vi "Poll Caller Idle.vi"(3 "error in (no error)":errorcluster, 4 "ExecAnchor in":refnum<class "ExecAnchor.lvclass">) -> (0 "error out":errorcluster, 1 "Caller Idle":bool)   [LabVIEW 2020, in "ExecAnchor.lvclass"]
uses:
  ExecAnchor.lvclass
  ExecAnchor.lvclass/ExecAnchor.ctl
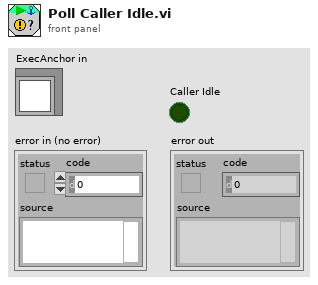
[diagram p1: front panel]
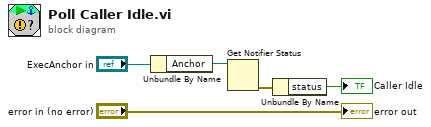
[diagram p0: block diagram]
diagram:
  n1 = Unbundle By Name("ExecAnchor in") -> ("Anchor"=w4:refnum<notifier>)
  n2 = Get Notifier Status(notifier=w4) -> (error out=w3:errorcluster)  [unwired: 1 in, 4 out]
  n3 = Unbundle By Name(w3) -> ("status"=→"Caller Idle":bool)
  "error out" <- "error in (no error)"
